vi "arrayI8.vi"(2 "Array In":i8[](array[numeric]), 3 "Base":i8) -> (0 "Array Out (not in place)":i8[](array[numeric]), 1 "Array Out":i8[](array[numeric]))   [LabVIEW 2012]
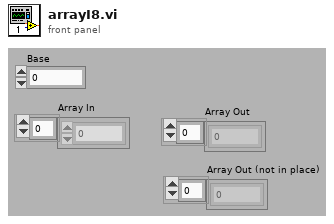
[diagram p1: front panel]
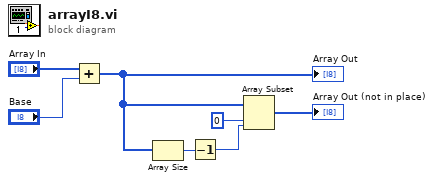
[diagram p0: block diagram]
diagram:
  n1 = Add(x="Array In", y="Base") -> (x+y=w2:i8[])
  "Array Out" <- w2
  n2 = Array Size(array=w2) -> (size(s)=w5:i32)
  n3 = Decrement(x=w5) -> (x-1=w6:i32)
  n4 = Array Subset(array=w2, index=0, length=w6) -> (→"Array Out (not in place)":i8[])
